vi "Plot individual and voting regression predictions.vi"() -> ()   [LabVIEW 2020]
doc: "A voting regressor is an ensemble meta-estimator that fits several base regressors, each on the whole dataset. Then it averages the individual predictions to form a final prediction. We will use three different regressors to predict the data: GradientBoostingRegressor, RandomForestRegressor, and LinearRegression). Then the above 3 regressors will be used for the VotingRegressor.\n\nFinally, we will plot the predictions made by all models for comparison.\n\nWe will work with the diabetes dataset which consists of 10 features collected from a cohort of diabetes patients. The target is a quantitative measure of disease progression one year after baseline."
uses:
  Model/Supervised/Ensemble/EnsembleRegressor/GradientBoostingRegressor/GradientBoostingRegressor.lvclass
  C:/Users/cipop/TDF Dropbox/2_Technologies de France/1 - Services et Etudes/PLAIY/2 - DEV/PLAIYLAB/code/Model/Model.lvclass
  C:/Users/cipop/TDF Dropbox/2_Technologies de France/1 - Services et Etudes/PLAIY/2 - DEV/PLAIYLAB/code/Model/Supervised/Ensemble/Ensemble.lvclass
  C:/Users/cipop/TDF Dropbox/2_Technologies de France/1 - Services et Etudes/PLAIY/2 - DEV/PLAIYLAB/code/Model/Supervised/Supervised.lvclass
  Model/Supervised/Ensemble/EnsembleRegressor/RandomForestRegressor/RandomForestRegressor.lvclass
  Model/Supervised/Linear_model/LinearRegressors/LinearRegression/LinearRegression.lvclass
  Model/Supervised/Ensemble/EnsembleRegressor/GradientBoostingRegressor/Controls/gradient_boosting_regressor_params.ctl
  Model/Supervised/Ensemble/EnsembleRegressor/RandomForestRegressor/Controls/random_forest_regressor_params.ctl
  Model/Supervised/Linear_model/LinearRegressors/LinearRegression/Controls/linear_regression_params.ctl
  Model/Supervised/Ensemble/EnsembleBlender/VotingRegressor/Controls/voting_regressor_params.ctl
  Model/Supervised/Supervised.lvclass
  Model/Supervised/Ensemble/EnsembleBlender/VotingRegressor/VotingRegressor.lvclass
  Model/Supervised/Ensemble/EnsembleRegressor/GradientBoostingRegressor/GradientBoostingRegressor.vi
  Model/Supervised/Ensemble/EnsembleRegressor/RandomForestRegressor/RandomForestRegressor.vi
  Model/Supervised/Linear_model/LinearRegressors/LinearRegression/LinearRegression.vi
  Model/Supervised/Ensemble/EnsembleBlender/VotingRegressor/VotingRegressor.vi
panel:
  out "Plot":dbl[][](graph)
  out "error out":errorcluster
  in  "error in":errorcluster
  in  "Local":T1
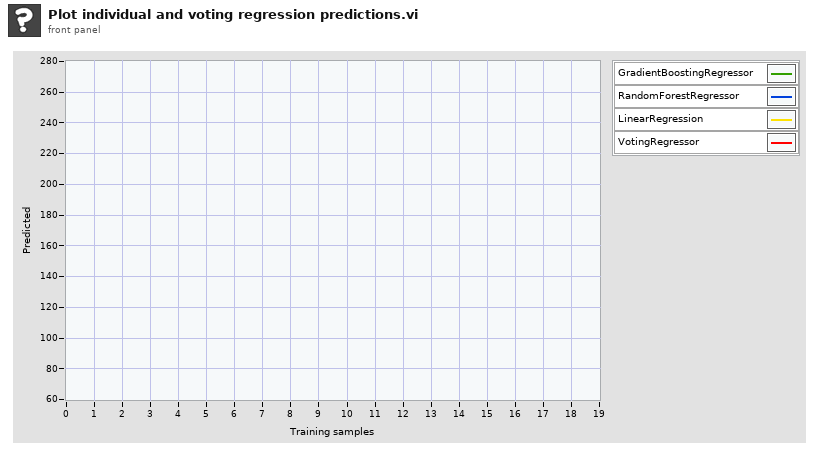
[diagram p1: front panel]
types:
  T1 = cluster{"X":dbl[][], "y":dbl[], "xt":dbl[][], "pred1":dbl[][], "pred2":dbl[][], "pred3":dbl[][], "pred4":dbl[][], "GradientBoostingRegressor":refnum<class "GradientBoostingRegressor.lvclass">, "RandomForestRegressor":refnum<class "RandomForestRegressor.lvclass">, "LinearRegression":refnum<class "LinearRegression.lvclass">}
  T2 = typedef "gradient_boosting_regressor_params.ctl" = cluster{"loss":string, "learning_rate":dbl, "n_estimators":dbl, "subsample":dbl, "criterion":string, "min_samples_split":dbl, "min_samples_leaf":dbl, "min_weight_fraction_leaf":dbl, "max_depth":dbl, "min_impurity_decrease":dbl, "init":string, "random_state":dbl, "max_features":cluster{"max_features_type":string, "max_features_float":dbl, "max_features_int":dbl}, "alpha":dbl, "verbose":dbl, "max_leaf_nodes":cluster{"max_leaf_nodes_type":string, "max_leaf_nodes_int":dbl}, "warm_start":bool, "validation_fraction":dbl, "n_iter_no_change":cluster{"n_iter_no_change_type":string, "n_iter_no_change_int":dbl}, "tol":dbl, "ccp_alpha":dbl}
  T3 = typedef "random_forest_regressor_params.ctl" = cluster{"n_estimators":dbl, "criterion":string, "max_depth":cluster{"max_depth_type":string, "max_depth_int":dbl}, "min_samples_split":dbl, "min_samples_leaf":dbl, "min_weight_fraction_leaf":dbl, "max_features":cluster{"max_features_type":string, "max_features_int":dbl, "max_features_float":dbl}, "max_leaf_nodes":cluster{"max_leaf_nodes_type":string, "max_leaf_nodes_int":dbl}, "min_impurity_decrease":dbl, "bootstrap":bool, "oob_score":bool, "n_jobs":dbl, "random_state":dbl, "verbose":dbl, "warm_start":bool, "ccp_alpha":dbl, "max_samples":cluster{"max_samples_type":string, "max_samples_int":dbl, "max_samples_float":dbl}}
  T4 = typedef "linear_regression_params.ctl" = cluster{"fit_intercept":bool, "normalize":bool, "copy_X":bool, "n_jobs":dbl, "positive":bool}
  T5 = typedef "voting_regressor_params.ctl" = cluster{"estimators":string[], "weights":cluster{"weights_type":string, "weights_list":dbl[]}, "n_jobs":dbl, "verbose":bool}
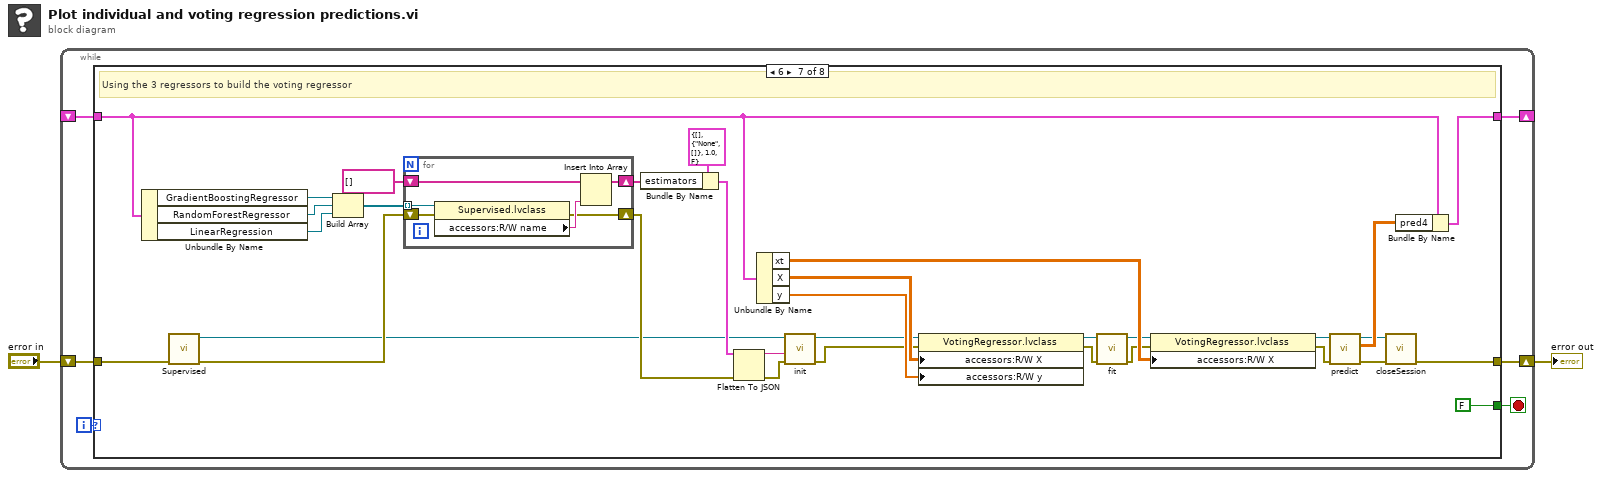
[diagram p0: block diagram]
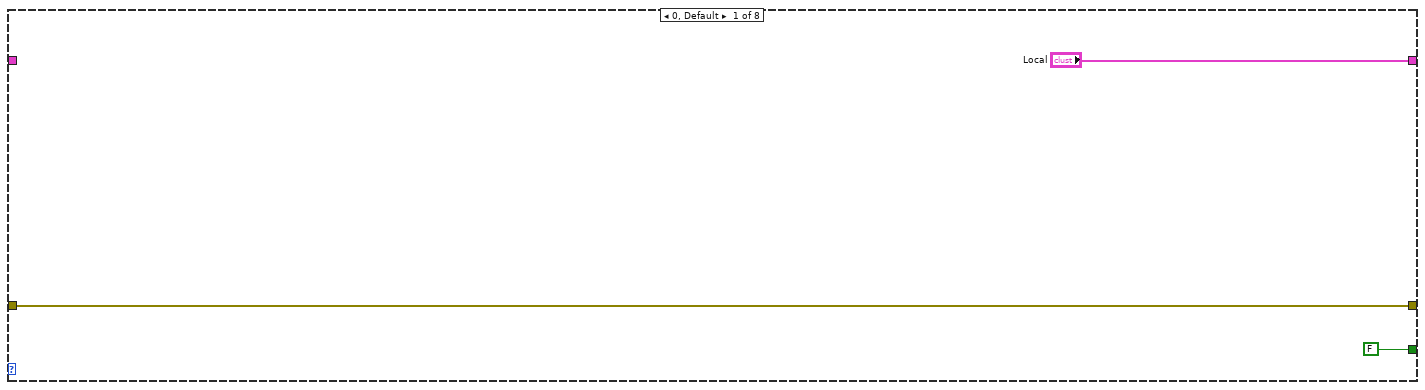
[diagram p2: hidden frame]
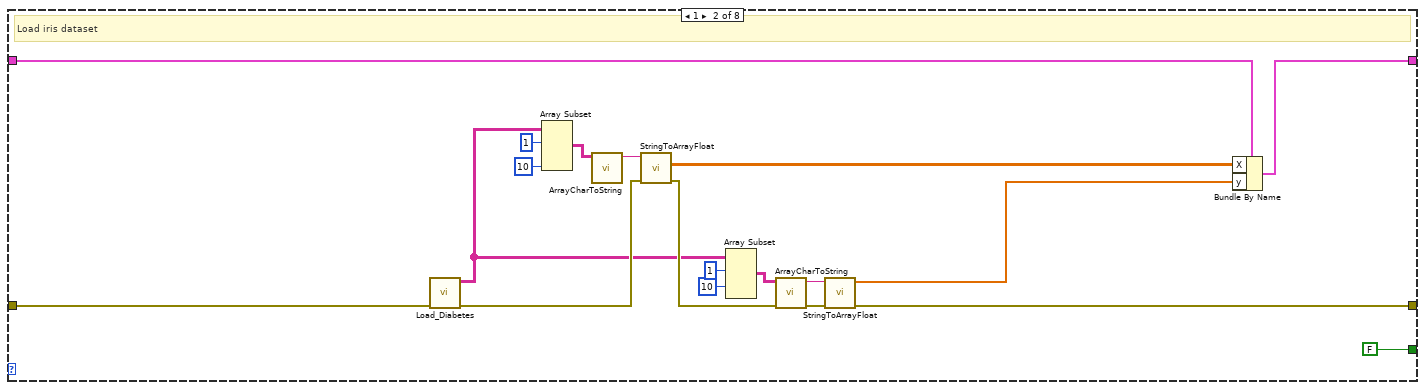
[diagram p3: hidden frame]
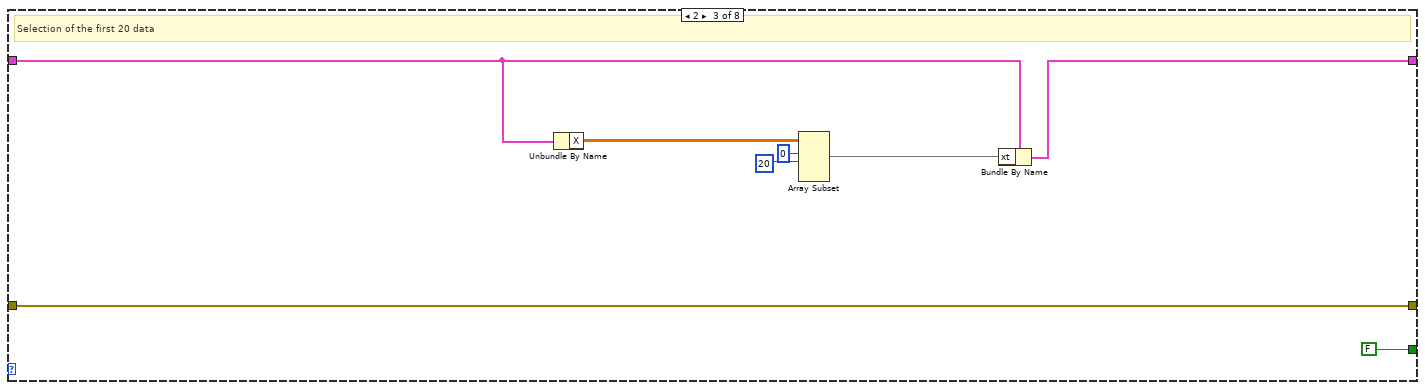
[diagram p4: hidden frame]
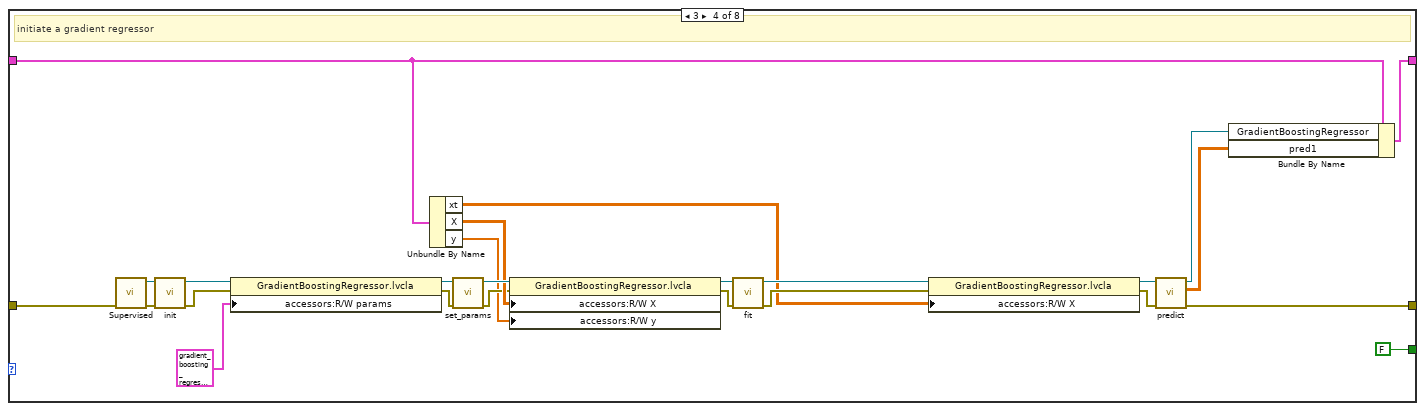
[diagram p5: hidden frame]
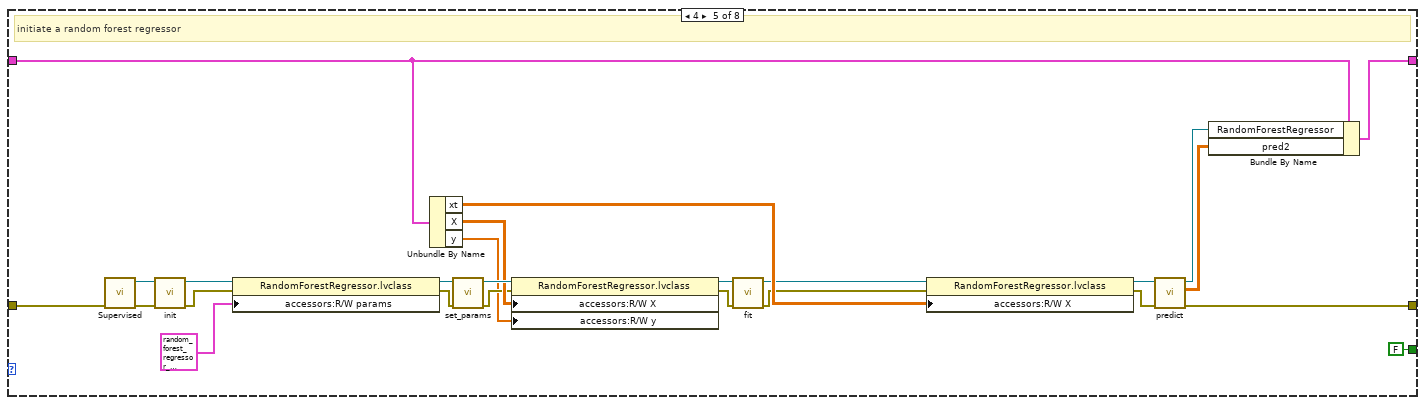
[diagram p6: hidden frame]
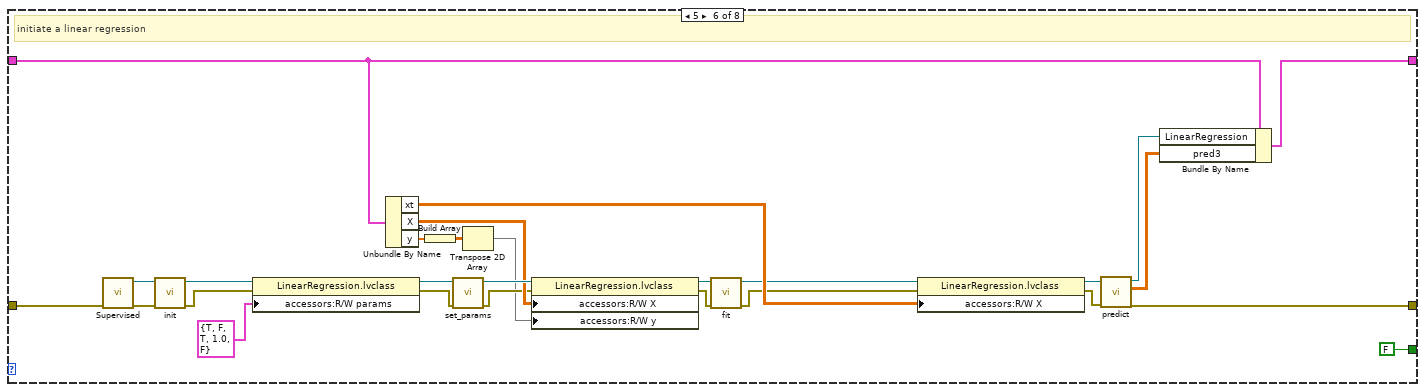
[diagram p7: hidden frame]
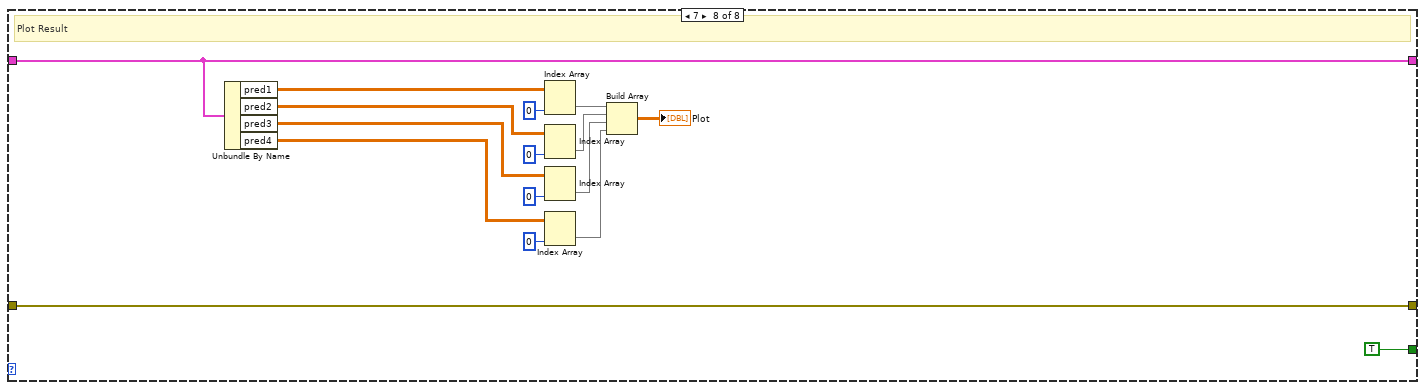
[diagram p8: hidden frame]
diagram:
  n1 = while {
    shift-right: [w6] -> w1
    shift-left: "error in" -> [w7]
    shift-right: [w5] -> _
    shift-left: _ -> [w4]
    i -> [w8]
    stop <- w3 stop-if-true
    n2 = case shown="6" w8 {
      tunnel: w7 -> [w10 w15 w37 w53 w72 w98 w146 w166]
      tunnel: [w10 w17 w37 w40 w64 w89 w130 w166] -> w6
      tunnel: ["Local" w12 w30 w38 w65 w102 w135 w167] -> w5
      tunnel: w4 -> [_ w28 w32 w47 w76 w103 w136 w167]
      tunnel: [FALSE FALSE FALSE FALSE FALSE FALSE FALSE TRUE] -> w3
      frame 0, Default {
      }
      frame 1 {
        # "Load iris dataset"
        n3 = call "Load_Diabetes.vi"("error in"=w15) -> ("error out"=w14:errorcluster, "Tableau"=w13:string[][])  [unwired: 9 in]
        n4 = Array Subset(array=w13, index (row)=1 ("index"), length (col)=10 ("length")) -> (w22:string[][])  [unwired: 2 in]
        n5 = call "ArrayCharToString.vi"("TAB"=w22) -> ("Instruction"=w23:string)  [unwired: 10 in]
        n6 = call "StringToArrayFloat.vi"("entrée d'erreur (pas d'erreur)"=w14, "Return value"=w23) -> ("error IO"=w18:errorcluster, "2DArray"=w19:dbl[][])  [unwired: 7 in, 1 out]
        n7 = Array Subset(array=w13, index (row)=1 ("index"), index (col)=10 ("index")) -> (w20:string[][])  [unwired: 2 in]
        n8 = call "ArrayCharToString.vi"("TAB"=w20) -> ("Instruction"=w21:string)  [unwired: 10 in]
        n9 = call "StringToArrayFloat.vi"("entrée d'erreur (pas d'erreur)"=w18, "Return value"=w21) -> ("error IO"=w17:errorcluster, "1DArray"=w16:dbl[])  [unwired: 7 in, 1 out]
        n10 = Bundle By Name(cluster=w28, "X"=w19, "y"=w16) -> (w12:T1)
      }
      frame 2 {
        # "Selection of the first 20 data"
        n11 = Unbundle By Name(w32) -> ("X"=w35:dbl[][])
        n12 = Array Subset(array=w35, index (row)=0 ("index"), length (row)=20 ("length")) -> (w31:dbl[][])  [unwired: 2 in]
        n13 = Bundle By Name(cluster=w32, "xt"=w31) -> (w30:T1)
      }
      frame 3 {
        # "initiate a gradient regressor"
        n14 = call-poly "Supervised.vi"("error in"=w53) -> ("error out"=w54:errorcluster, "out"=w55:refnum<class "GradientBoostingRegressor.lvclass">)  [unwired: 9 in]
        n15 = call-dynamic "init.vi"("error in (no error)"=w54, "Model en entrée"=w55) -> ("error out"=w58:errorcluster, "Model en sortie"=w61:refnum<class "GradientBoostingRegressor.lvclass">)  [unwired: 8 in]
        n16 = property class="GradientBoostingRegressor.lvcla"(reference=w61, error in=w58, "accessors:R/W params"=T2 {"loss"="ls", "learning_rate"=0.1, "n_estimators"=100.0, "subsample"=1.0, "criterion"="friedman_mse", "min_samples_split"=2.0, "min_samples_leaf"=1.0, "min_weight_fraction_leaf"=0.0, "max_depth"=3.0, "min_impurity_decrease"=0.0, "init"="None", "random_state"=1.0, "max_features"={"max_features_type"="None", "max_features_float"=1.0, "max_features_int"=0.0}, "alpha"=0.9, "verbose"=0.0, "max_leaf_nodes"={"max_leaf_nodes_type"="None", "max_leaf_nodes_int"=0.0}, "warm_start"=FALSE, "validation_fraction"=0.1, "n_iter_no_change"={"n_iter_no_change_type"="None", "n_iter_no_change_int"=0.0}, "tol"=0.0001, "ccp_alpha"=0.0} ("R/W params")) -> (reference out=w60:refnum<class "GradientBoostingRegressor.lvclass">, error out=w51:errorcluster)
        n17 = Unbundle By Name(w47) -> ("xt"=w43:dbl[][], "X"=w57:dbl[][], "y"=w49:dbl[])
        n18 = call-dynamic "set_params.vi"("error in (no error)"=w51, "GradientBoostingRegressor.lvclass 2"=w60) -> ("error out"=w50:errorcluster, "GradientBoostingRegressor.lvclass"=w59:refnum<class "GradientBoostingRegressor.lvclass">)  [unwired: 8 in]
        n19 = property class="GradientBoostingRegressor.lvcla"(reference=w59, error in=w50, "accessors:R/W X"=w57, "accessors:R/W y"=w49) -> (reference out=w56:refnum<class "GradientBoostingRegressor.lvclass">, error out=w48:errorcluster)
        n20 = call-dynamic "fit.vi"("error in (no error)"=w48, "Ensemble.lvclass 2"=w56) -> ("error out"=w44:errorcluster, "Ensemble.lvclass"=w45:refnum<class "GradientBoostingRegressor.lvclass">)  [unwired: 8 in]
        n21 = property class="GradientBoostingRegressor.lvcla"(reference=w45, error in=w44, "accessors:R/W X"=w43) -> (reference out=w41:refnum<class "GradientBoostingRegressor.lvclass">, error out=w42:errorcluster)
        n22 = call-dynamic "predict.vi"("error in (no error)"=w42, "Ensemble.lvclass 2"=w41) -> ("error out"=w40:errorcluster, "C"=w46:dbl[][], "Ensemble.lvclass"=w39:refnum<class "GradientBoostingRegressor.lvclass">)  [unwired: 7 in]
        n23 = Bundle By Name(cluster=w47, "GradientBoostingRegressor"=w39, "pred1"=w46) -> (w38:T1)
      }
      frame 4 {
        # "initiate a random forest regressor"
        n24 = call-poly "Supervised.vi"("error in"=w72) -> ("error out"=w73:errorcluster, "out"=w74:refnum<class "RandomForestRegressor.lvclass">)  [unwired: 9 in]
        n25 = call-dynamic "init.vi"("error in (no error)"=w73, "Model en entrée"=w74) -> ("error out"=w83:errorcluster, "Model en sortie"=w86:refnum<class "RandomForestRegressor.lvclass">)  [unwired: 8 in]
        n26 = property class="RandomForestRegressor.lvclass"(reference=w86, error in=w83, "accessors:R/W params"=T3 {"n_estimators"=100.0, "criterion"="mse", "max_depth"={"max_depth_type"="None", "max_depth_int"=0.0}, "min_samples_split"=2.0, "min_samples_leaf"=1.0, "min_weight_fraction_leaf"=0.0, "max_features"={"max_features_type"="None", "max_features_int"=0.0, "max_features_float"=0.0}, "max_leaf_nodes"={"max_leaf_nodes_type"="None", "max_leaf_nodes_int"=100.0}, "min_impurity_decrease"=0.0, "bootstrap"=TRUE, "oob_score"=FALSE, "n_jobs"=1.0, "random_state"=1.0, "verbose"=0.0, "warm_start"=FALSE, "ccp_alpha"=0.0, "max_samples"={"max_samples_type"="None", "max_samples_int"=0.0, "max_samples_float"=0.0}} ("R/W params")) -> (reference out=w85:refnum<class "RandomForestRegressor.lvclass">, error out=w80:errorcluster)
        n27 = Unbundle By Name(w76) -> ("xt"=w70:dbl[][], "X"=w82:dbl[][], "y"=w78:dbl[])
        n28 = call-dynamic "set_params.vi"("error in (no error)"=w80, "RandomForestRegressor.lvclass 2"=w85) -> ("error out"=w79:errorcluster, "RandomForestRegressor.lvclass"=w84:refnum<class "RandomForestRegressor.lvclass">)  [unwired: 8 in]
        n29 = property class="RandomForestRegressor.lvclass"(reference=w84, error in=w79, "accessors:R/W X"=w82, "accessors:R/W y"=w78) -> (reference out=w81:refnum<class "RandomForestRegressor.lvclass">, error out=w77:errorcluster)
        n30 = call-dynamic "fit.vi"("error in (no error)"=w77, "Ensemble.lvclass 2"=w81) -> ("error out"=w68:errorcluster, "Ensemble.lvclass"=w69:refnum<class "RandomForestRegressor.lvclass">)  [unwired: 8 in]
        n31 = property class="RandomForestRegressor.lvclass"(reference=w69, error in=w68, "accessors:R/W X"=w70) -> (reference out=w67:refnum<class "RandomForestRegressor.lvclass">, error out=w66:errorcluster)
        n32 = call-dynamic "predict.vi"("error in (no error)"=w66, "Ensemble.lvclass 2"=w67) -> ("error out"=w64:errorcluster, "C"=w75:dbl[][], "Ensemble.lvclass"=w63:refnum<class "RandomForestRegressor.lvclass">)  [unwired: 7 in]
        n33 = Bundle By Name(cluster=w76, "RandomForestRegressor"=w63, "pred2"=w75) -> (w65:T1)
      }
      frame 5 {
        # "initiate a linear regression"
        n34 = call-poly "Supervised.vi"("error in"=w98) -> ("error out"=w99:errorcluster, "out"=w100:refnum<class "LinearRegression.lvclass">)  [unwired: 9 in]
        n35 = call-dynamic "init.vi"("error in (no error)"=w99, "Model en entrée"=w100) -> ("error out"=w110:errorcluster, "Model en sortie"=w113:refnum<class "LinearRegression.lvclass">)  [unwired: 8 in]
        n36 = property class="LinearRegression.lvclass"(reference=w113, error in=w110, "accessors:R/W params"=T4 {"fit_intercept"=TRUE, "normalize"=FALSE, "copy_X"=TRUE, "n_jobs"=1.0, "positive"=FALSE} ("R/W params")) -> (reference out=w112:refnum<class "LinearRegression.lvclass">, error out=w107:errorcluster)
        n37 = Unbundle By Name(w103) -> ("xt"=w94:dbl[][], "X"=w109:dbl[][], "y"=w105:dbl[])
        n38 = Build Array(w105) -> (w97:dbl[][])
        n39 = call-dynamic "set_params.vi"("error in (no error)"=w107, "LinearRegression.lvclass 2"=w112) -> ("error out"=w106:errorcluster, "LinearRegression.lvclass"=w111:refnum<class "LinearRegression.lvclass">)  [unwired: 8 in]
        n40 = Transpose 2D Array(2D array=w97) -> (transposed array=w96:dbl[][])
        n41 = property class="LinearRegression.lvclass"(reference=w111, error in=w106, "accessors:R/W X"=w109, "accessors:R/W y"=w96) -> (reference out=w108:refnum<class "LinearRegression.lvclass">, error out=w104:errorcluster)
        n42 = call-dynamic "fit.vi"("error in (no error)"=w104, "LinearRegression.lvclass 2"=w108) -> ("error out"=w92:errorcluster, "LinearRegression.lvclass"=w93:refnum<class "LinearRegression.lvclass">)  [unwired: 8 in]
        n43 = property class="LinearRegression.lvclass"(reference=w93, error in=w92, "accessors:R/W X"=w94) -> (reference out=w91:refnum<class "LinearRegression.lvclass">, error out=w90:errorcluster)
        n44 = call-dynamic "predict.vi"("error in (no error)"=w90, "LinearRegression.lvclass 2"=w91) -> ("error out"=w89:errorcluster, "C"=w101:dbl[][], "LinearRegression.lvclass"=w88:refnum<class "LinearRegression.lvclass">)  [unwired: 7 in]
        n45 = Bundle By Name(cluster=w103, "LinearRegression"=w88, "pred3"=w101) -> (w102:T1)
      }
      frame 6 {
        # "Using the 3 regressors to build the voting regressor"
        n46 = Unbundle By Name(w136) -> ("GradientBoostingRegressor"=w143:refnum<class "GradientBoostingRegressor.lvclass">, "RandomForestRegressor"=w141:refnum<class "RandomForestRegressor.lvclass">, "LinearRegression"=w140:refnum<class "LinearRegression.lvclass">)
        n47 = call-poly "Supervised.vi"("error in"=w146) -> ("error out"=w124:errorcluster, "out"=w118:refnum<class "VotingRegressor.lvclass">)  [unwired: 9 in]
        n48 = Build Array(w143, w141, w140) -> (w144:refnum<class "Supervised.lvclass">[])
        n49 = for {
          tunnel: w144 -> [w149] mode=indexing
          shift-right: [w150] -> w125
          shift-left: string[] [] -> [w152]
          shift-right: [w147] -> w120
          shift-left: w124 -> [w148]
          n50 = property class="Supervised.lvclass"(reference=w149, error in=w148) -> (error out=w147:errorcluster, "accessors:R/W name"=w151:string)  [unwired: 1 out]
          n51 = Insert Into Array(array=w152, new element=w151) -> (w150:string[])  [unwired: 1 in]
        }
        n52 = Bundle By Name(cluster=T5 {"estimators"=[], "weights"={"weights_type"="None", "weights_list"=[]}, "n_jobs"=1.0, "verbose"=FALSE} ("R/W params"), "estimators"=w125) -> (w123:T5)
        n53 = Flatten To JSON(anything=w123, error in (no error)=w120) -> (JSON string=w115:string, 11:w116:errorcluster)  [unwired: 1 in]
        n54 = Unbundle By Name(w136) -> ("xt"=w139:dbl[][], "X"=w138:dbl[][], "y"=w137:dbl[])
        n55 = call-dynamic "init.vi"("error in (no error)"=w116, "json of params"=w115, "EnsembleBlender in"=w118) -> ("error out"=w117:errorcluster, "EnsembleBlender out"=w119:refnum<class "VotingRegressor.lvclass">)  [unwired: 7 in]
        n56 = property class="VotingRegressor.lvclass"(reference=w119, error in=w117, "accessors:R/W X"=w138, "accessors:R/W y"=w137) -> (reference out=w128:refnum<class "VotingRegressor.lvclass">, error out=w129:errorcluster)
        n57 = call-dynamic "fit.vi"("error in (no error)"=w129, "Ensemble.lvclass 2"=w128) -> ("error out"=w121:errorcluster, "Ensemble.lvclass"=w122:refnum<class "VotingRegressor.lvclass">)  [unwired: 8 in]
        n58 = property class="VotingRegressor.lvclass"(reference=w122, error in=w121, "accessors:R/W X"=w139) -> (reference out=w126:refnum<class "VotingRegressor.lvclass">, error out=w127:errorcluster)
        n59 = call-dynamic "predict.vi"("error in (no error)"=w127, "Ensemble.lvclass 2"=w126) -> ("error out"=w131:errorcluster, "C"=w134:dbl[][], "Ensemble.lvclass"=w132:refnum<class "VotingRegressor.lvclass">)  [unwired: 7 in]
        n60 = call-dynamic "closeSession.vi"("error in"=w131, "Python en entrée"=w132) -> ("error out"=w130:errorcluster)  [unwired: 8 in, 1 out]
        n61 = Bundle By Name(cluster=w136, "pred4"=w134) -> (w135:T1)
      }
      frame 7 {
        # "Plot Result"
        n62 = Unbundle By Name(w167) -> ("pred1"=w165:dbl[][], "pred2"=w160:dbl[][], "pred3"=w158:dbl[][], "pred4"=w154:dbl[][])
        n63 = Index Array(array=w165, index (col)=0 ("disabled index (col)")) -> (element=w163:dbl[])  [unwired: 1 in]
        n64 = Index Array(array=w160, index (col)=0 ("disabled index (col)")) -> (element=w157:dbl[])  [unwired: 1 in]
        n65 = Index Array(array=w158, index (col)=0 ("disabled index (col)")) -> (element=w156:dbl[])  [unwired: 1 in]
        n66 = Index Array(array=w154, index (col)=0 ("disabled index (col)")) -> (element=w153:dbl[])  [unwired: 1 in]
        n67 = Build Array(w163, w157, w156, w153) -> (→"Plot":dbl[][])
      }
    }
  }
  "error out" <- w1
